vi "TCP Engine JSON to LV Data.vi"(8 "error in":errorcluster, 11 "Cmd String":string) -> (0 "error out":errorcluster, 1 "SubCmd":string, 2 "Command":string, 3 "Interface":string, 4 "Data":variant, 5 "Data":string)   [LabVIEW 2024, in "TCP Engine.lvlib"]
doc: "All Rights Reserved © 2017 SyncSols"
uses:
  TCP Engine.lvlib
  Host-Control's/TCP Tx-Rx cluster.ctl
  <vilib>/addons/_JKI.lib/Serialization/JSON/JKI JSON Serialization.lvlib
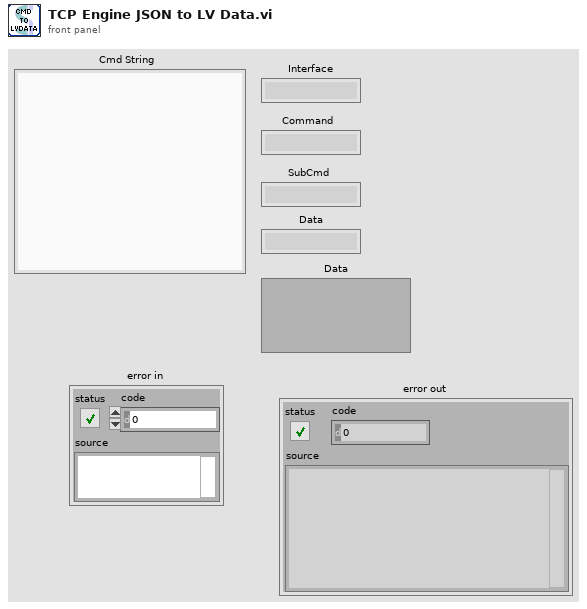
[diagram p1: front panel]
types:
  T1 = typedef "TCP Tx-Rx cluster.ctl" = cluster{"Interface":string, "Command":string, "SubCmd":string, "Data":variant}
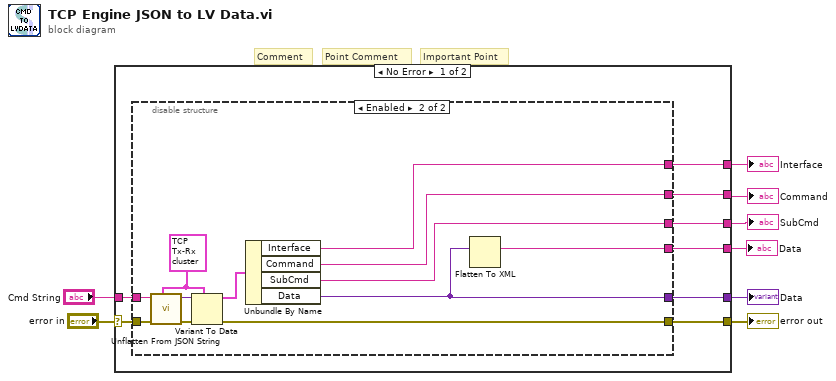
[diagram p0: block diagram]
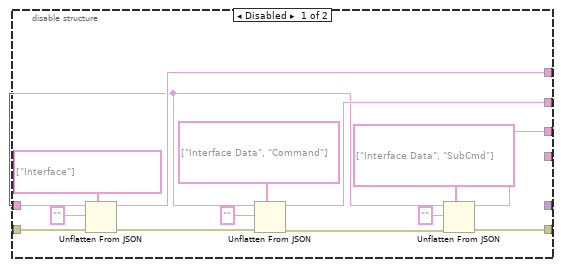
[diagram p2: hidden frame]
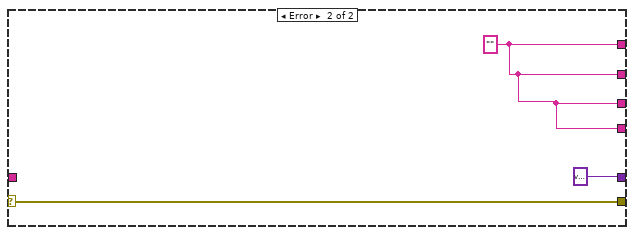
[diagram p3: hidden frame]
diagram:
  # "Important Point"
  # "Point Comment"
  # "Comment"
  n1 = case shown="No Error" "error in" {
    selector: "error in" -> [w16 w45]
    tunnel: [w13 w45] -> w8
    tunnel: "Cmd String" -> [w11 _]
    tunnel: [w12 w43] -> w5
    tunnel: [w14 w43] -> w4
    tunnel: [w15 w43] -> w3
    tunnel: [w10 variant ("Data")] -> w2
    tunnel: [w9 w43] -> w1
    frame No Error {
      n2 = disable-structure shown="Enabled" {
        disable-tunnel: w16 -> [w30 w36]
        disable-tunnel: [w25 w42] -> w15
        disable-tunnel: [w23 w41] -> w14
        disable-tunnel: [w19 w32] -> w13
        disable-tunnel: [w18 w40] -> w12
        disable-tunnel: w11 -> [w17 w37]
        disable-tunnel: [_ w39] -> w10
        disable-tunnel: [_ w38] -> w9
        frame Disabled {
          n3 = Unflatten From JSON(path=string[] ["Interface"], JSON string=w17, type and defaults="", error in (no error)=w30) -> (value=w25:string, error out=w27:errorcluster)  [unwired: 3 in]
          n4 = Unflatten From JSON(path=string[] ["Interface Data", "Command"], JSON string=w17, type and defaults="", error in (no error)=w27) -> (value=w23:string, error out=w20:errorcluster)  [unwired: 3 in]
          n5 = Unflatten From JSON(path=string[] ["Interface Data", "SubCmd"], JSON string=w17, type and defaults="", error in (no error)=w20) -> (value=w18:string, error out=w19:errorcluster)  [unwired: 3 in]
        }
        frame Enabled {
          w34 = T1 {"Interface"="CPU", "Command"="CPU Info", "SubCmd"="Monitor", "Data"=variant} ("TCP Tx-Rx Cluster")
          n6 = call <vilib>:"Unflatten From JSON String.vi"("Type and Defaults"=w34, "error in"=w36, "JSON String"=w37) -> ("error out"=w33:errorcluster, "Variant"=w35:variant)  [unwired: 7 in]
          n7 = Variant To Data(error in=w33, type=w34, Variant=w35) -> (data=w31:T1, error out=w32:errorcluster)
          n8 = Unbundle By Name(w31) -> ("Interface"=w42:string, "Command"=w41:string, "SubCmd"=w40:string, "Data"=w39:variant)
          n9 = Flatten To XML(anything=w39) -> (xml string=w38:string)
        }
      }
    }
    frame Error {
      w43 = ""
    }
  }
  "error out" <- w8
  "SubCmd" <- w5
  "Command" <- w4
  "Interface" <- w3
  "Data" <- w2
  "Data" <- w1
